vi "SMUSineWithReferenceTrigger.vi"() -> ()   [LabVIEW 2023]
uses:
  <instrlib>/niDCPower/nidcpower.llb/niDCPower Source Mode.ctl
  <instrlib>/niDCPower/nidcpower.llb/niDCPower Output Function.ctl
  <instrlib>/niDCPower/nidcpower.llb/niDCPower Sequence Attribute Type.ctl
  <instrlib>/niDCPower/nidcpower.llb/niDCPower Create Advanced Sequence Step With Channels.vi
  <instrlib>/niScope/Measurements/niScope Fetch Array Measurement Cluster.vi
  <instrlib>/niDCPower/nidcpower.llb/niDCPower Export Signal - Signal.ctl
  <instrlib>/niScope/Configure/Trigger/niScope Configure Trigger Digital.vi
  <instrlib>/niScope/Controls/niScope trigger source digital.ctl
  <instrlib>/niScope/Controls/niScope trigger slope.ctl
  <instrlib>/niScope/Controls/niScope vertical coupling.ctl
panel:
  in  "Configure":enum32{"SMU", "Scope"}(tab)
  in  "SMUname":refnum<k15> caption="resource name"
  in  "DC offset":dbl
  in  "Amplitude":dbl
  in  "Frequency":dbl format="%#_6p"
  in  "Samples per Sine":u16
  in  "?":enum32{"Standard Transients", "Custom"}(tab)
  in  "Source:Transient Response":i32(ring)=1041 items=["Slow"=1041, "Normal"=1038, "Fast"=1039, "Custom"=1042]
  in  "Gain Bandwidth":dbl=5000.0
  in  "Pole-Zero Ratio":dbl=0.16
  in  "Compensation Frequency":dbl=50000.0
  in  "Fixed Source Delay of":dbl format="%#_6p"
  in  "Amount of Sine Swings":i32
  out "Apperature Time":dbl format="%#_6p"
  in  "resource name":refnum<k15> caption="Scope Name"
  in  "Scope sample rate":dbl=20000000.0 caption="min sample rate" format="%^.2e"
  in  "number of records":i32=1
  in  "min record length":i32=1000
  in  "vertical coupling":T1=1 items=["AC", "DC", "Ground"]
  in  "channels":string="0"
  out "Stimulus In":cluster{dbl, dbl}[](graph)
  out "SMU Voltage Out":cluster{dbl, dbl}[](graph)
  out "error out":errorcluster
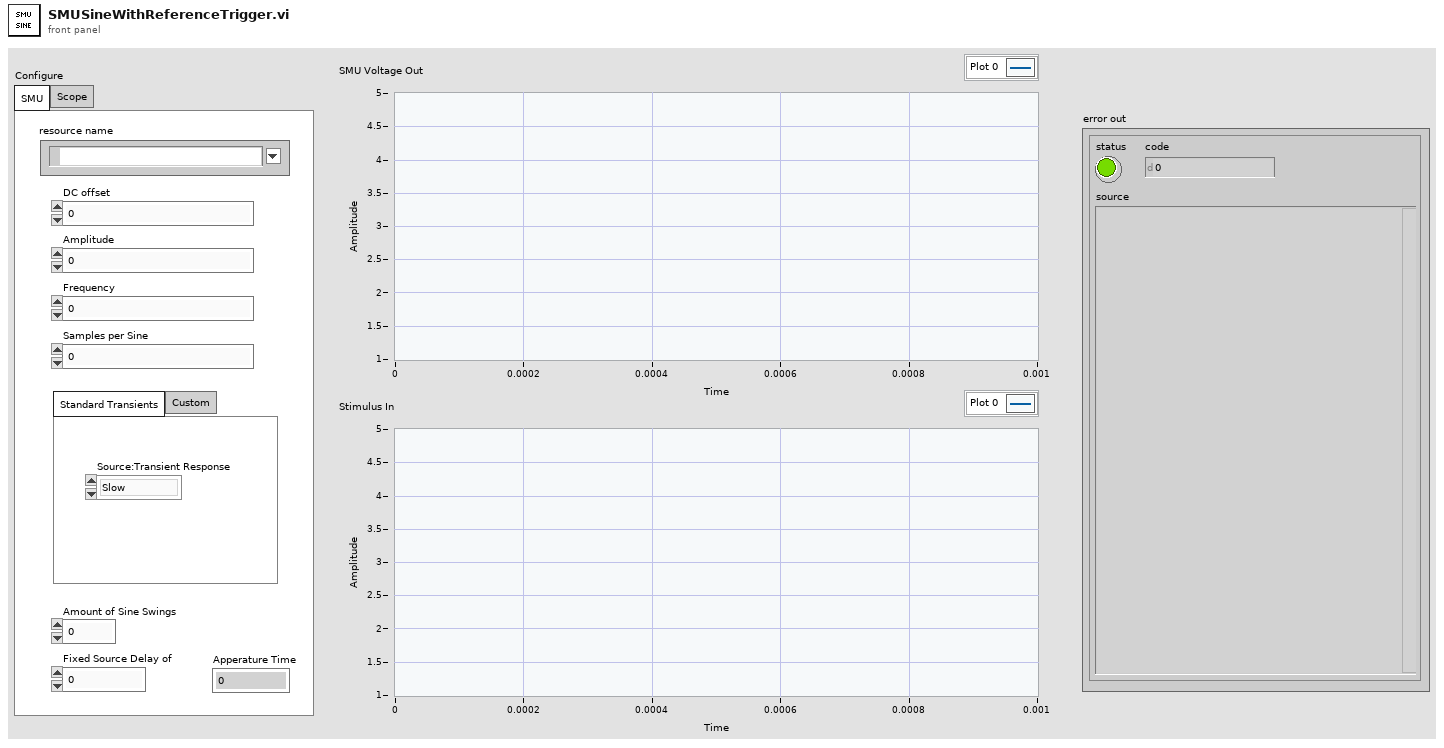
[diagram p1: front panel]
types:
  T1 = typedef "niScope vertical coupling.ctl" = i32
  T2 = typedef "niScope trigger slope.ctl" = i32
  T3 = typedef "niScope trigger source digital.ctl" = string
  T4 = typedef "niDCPower Export Signal - Signal.ctl" = i32
  T5 = typedef "niDCPower Output Function.ctl" = i32
  T6 = typedef "niDCPower Source Mode.ctl" = i32
  T7 = typedef "niDCPower Sequence Attribute Type.ctl" = i32
  T8 = cluster{"relativeInitialX":dbl, "xIncrement":dbl, "measWfm":dbl[]}
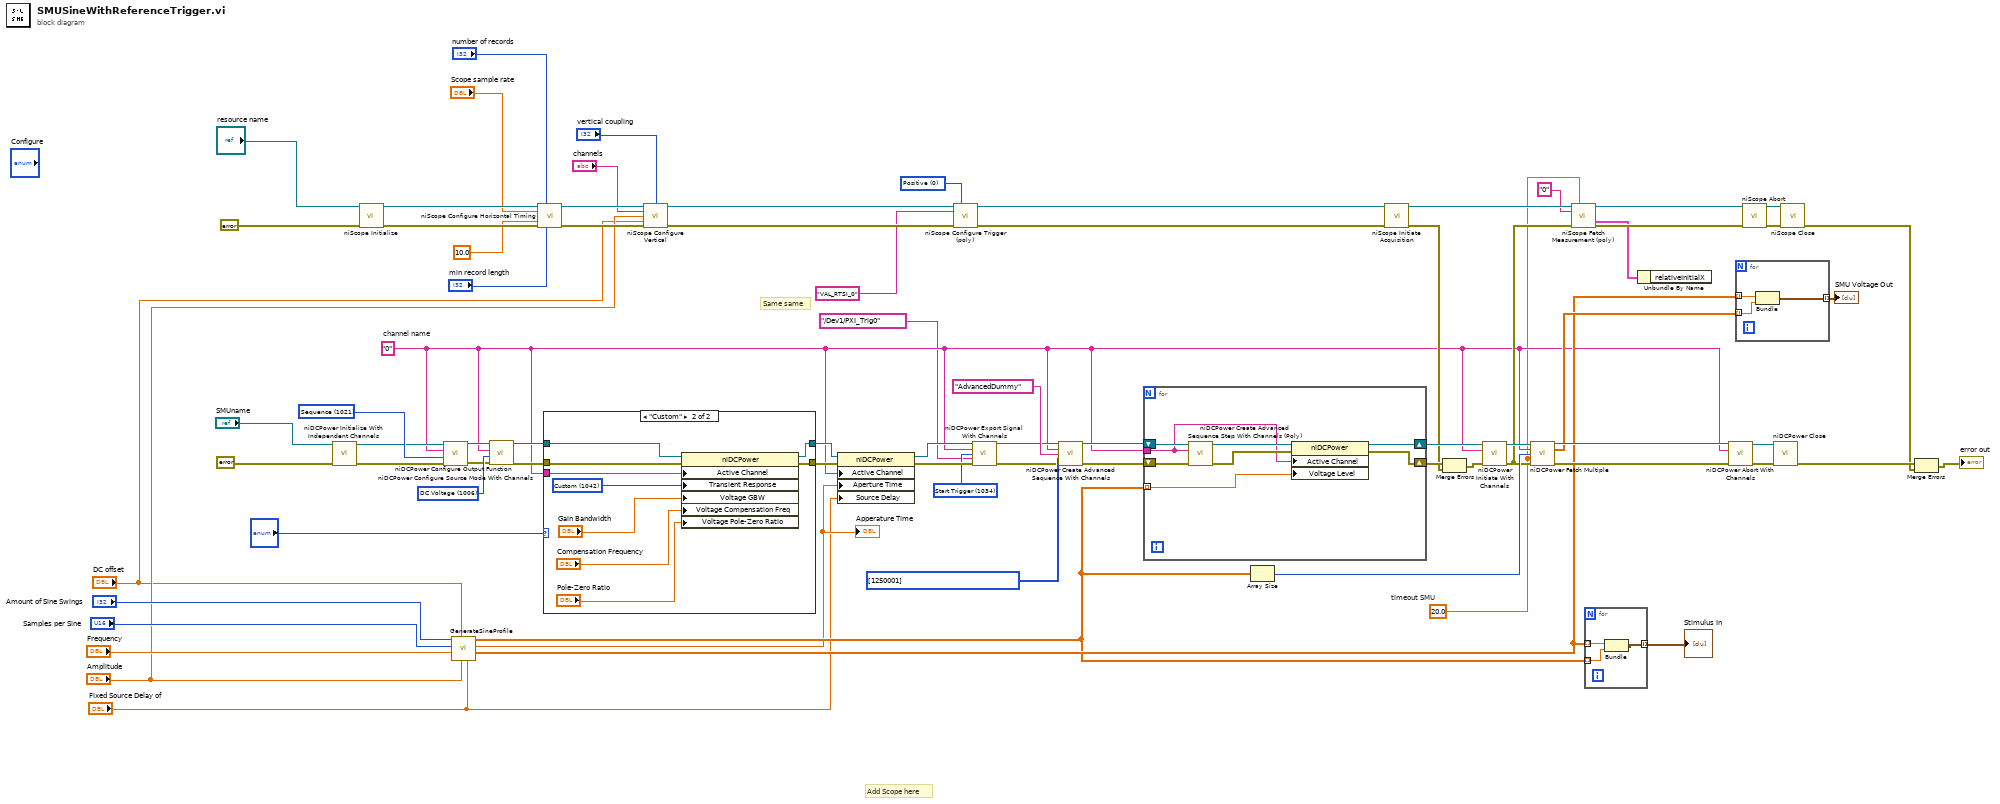
[diagram p0: block diagram]
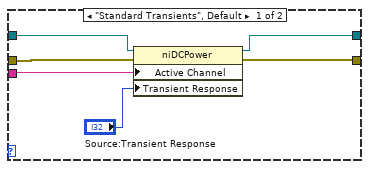
[diagram p2: hidden frame]
diagram:
  w3 = T2 0 items=["Positive", "Negative"] ("trigger slope")
  w6 = T4 1034 items=["Source Complete Event"=1030, "Measure Complete Event"=1031, "Sequence Iteration Complete Event"=1032, "Sequence Engine Done Event"=1033, "Pulse Complete Event"=1051, "Ready For Pulse Trigger Event"=1052, "Start Trigger"=1034, "Source Trigger"=1035, "Measure Trigger"=1036, "Sequence Advance Trigger"=1037, "Pulse Trigger"=1053] ("signal")
  w2 = 20.0  # timeout SMU
  w63 = T5 1006 items=["DC Voltage"=1006, "DC Current"=1007, "Pulse Voltage"=1049, "Pulse Current"=1050] ("output function")
  w66 = T6 1021 items=["Single Point"=1020, "Sequence"=1021] ("source mode")
  w67 = T7[] [1250001] items=["Source -> Output Function"=1150008, "Source -> Output Enabled"=1250006, "Source -> Output Resistance"=1150061, "Source -> Transient Response"=1150062, "Source -> Custom Transient Response -> Voltage Gain Bandwidth"=1150067, "Source -> Custom Transient Response -> Voltage Compensation Frequency"=1150068, "Source -> Custom Transient Response -> Voltage Pole-Zero Ratio"=1150069, "Source -> Custom Transient Response -> Current Gain Bandwidth"=1150070, "Source -> Custom Transient Response -> Current Compensation Frequency"=1150071, "Source -> Custom Transient Response -> Current Pole-Zero Ratio"=1150072, "Source -> DC Voltage -> Voltage Level"=1250001, "Source -> DC Voltage -> Voltage Level Range"=1150005, "Source -> DC Voltage -> Current Limit"=1250005, "Source -> DC Voltage -> Current Limit High"=1150187, "Source -> DC Voltage -> Current Limit Low"=1150188, "Source -> DC Voltage -> Current Limit Range"=1150004, "Source -> DC Current -> Current Level"=1150009, "Source -> DC Current -> Current Level Range"=1150011, "Source -> DC Current -> Voltage Limit"=1150010, "Source -> DC Current -> Voltage Limit High"=1150185, "Source -> DC Current -> Voltage Limit Low"=1150186, "Source -> DC Current -> Voltage Limit Range"=1150012, "Source -> DC Current -> Current Level Slew Rate -> Rising"=1150343, "Source -> DC Current -> Current Level Slew Rate -> Falling"=1150344, "Source -> Pulse Voltage -> Pulse Voltage Level"=1150080, "Source -> Pulse Voltage -> Pulse Bias Voltage Level"=1150082, "Source -> Pulse Voltage -> Pulse Voltage Level Range"=1150084, "Source -> Pulse Voltage -> Pulse Current Limit"=1150081, "Source -> Pulse Voltage -> Pulse Current Limit High"=1150193, "Source -> Pulse Voltage -> Pulse Current Limit Low"=1150194, "Source -> Pulse Voltage -> Pulse Bias Current Limit"=1150083, "Source -> Pulse Voltage -> Pulse Bias Current Limit High"=1150195, "Source -> Pulse Voltage -> Pulse Bias Current Limit Low"=1150196, "Source -> Pulse Voltage -> Pulse Current Limit Range"=1150085, "Source -> Pulse Current -> Pulse Current Level"=1150086, "Source -> Pulse Current -> Pulse Bias Current Level"=1150088, "Source -> Pulse Current -> Pulse Current Level Range"=1150090, "Source -> Pulse Current -> Pulse Voltage Limit"=1150087, "Source -> Pulse Current -> Pulse Voltage Limit High"=1150189, "Source -> Pulse Current -> Pulse Voltage Limit Low"=1150190, "Source -> Pulse Current -> Pulse Bias Voltage Limit"=1150089, "Source -> Pulse Current -> Pulse Bias Voltage Limit High"=1150191, "Source -> Pulse Current -> Pulse Bias Voltage Limit Low"=1150192, "Source -> Pulse Current -> Pulse Voltage Limit Range"=1150091, "Source -> Advanced -> Source Delay"=1150051, "Source -> Advanced -> Pulse Bias Delay"=1150092, "Source -> Advanced -> Pulse On Time"=1150093, "Source -> Advanced -> Pulse Off Time"=1150094, "Source -> Advanced -> OVP Enabled"=1250002, "Source -> Advanced -> OVP Limit"=1250003, "Source -> Advanced -> Compliance Limit Symmetry"=1150184, "Source -> Advanced -> Sequence Step Delta Time"=1150198, "Source -> Advanced -> Conduction Voltage -> Mode"=1150350, "Source -> Advanced -> Conduction Voltage -> On Threshold"=1150351, "Source -> Advanced -> Conduction Voltage -> Off Threshold"=1150352, "Measurement -> Sense"=1150013, "Measurement -> Aperture Time"=1150058, "Measurement -> Measure Record Length"=1150063, "Measurement -> Advanced -> DC Noise Rejection"=1150066, "Measurement -> Autorange"=1150244, "Measurement -> Advanced -> Autorange Behavior"=1150245, "Measurement -> Advanced -> Autorange Aperture Time Mode"=1150246, "Measurement -> Advanced -> Autorange Minimum Aperture Time"=1150247, "Measurement -> Advanced -> Autorange Minimum Aperture Time Units"=1150248, "Measurement -> Advanced -> Autorange Minimum Current Range"=1150255, "Measurement -> Advanced -> Autorange Minimum Voltage Range"=1150256, "Measurement -> Advanced -> Autorange Threshold Mode"=1150257, "Measurement -> Advanced -> Autorange Maximum Delay After Range Change"=1150322, "LCR -> Instrument Mode"=1150208, "LCR -> Source Delay Mode"=1150315, "LCR -> Measurement Time"=1150218, "LCR -> Custom Measurement Time"=1150258, "LCR -> AC Stimulus -> Function"=1150209, "LCR -> AC Stimulus -> Frequency"=1150210, "LCR -> AC Stimulus -> Voltage Amplitude"=1150211, "LCR -> AC Stimulus -> Current Amplitude"=1150212, "LCR -> AC Stimulus -> Advanced -> Voltage Range"=1150265, "LCR -> AC Stimulus -> Advanced -> Current Range"=1150267, "LCR -> AC Stimulus -> Advanced -> Source Aperture Time"=1150349, "LCR -> DC Bias -> Source"=1150213, "LCR -> DC Bias -> Voltage Level"=1150214, "LCR -> DC Bias -> Current Level"=1150215, "LCR -> DC Bias -> Advanced -> Voltage Range"=1150266, "LCR -> DC Bias -> Advanced -> Current Range"=1150274, "LCR -> DC Bias -> Advanced -> Transient Response"=1150347, "LCR -> Compensation -> Open -> Enabled"=1150220, "LCR -> Compensation -> Open -> Conductance"=1150261, "LCR -> Compensation -> Open -> Susceptance"=1150262, "LCR -> Compensation -> Short -> Enabled"=1150221, "LCR -> Compensation -> Short -> Resistance"=1150263, "LCR -> Compensation -> Short -> Reactance"=1150264, "LCR -> Compensation -> Load -> Enabled"=1150222, "LCR -> Compensation -> Load -> Measured Resistance"=1150268, "LCR -> Compensation -> Load -> Measured Reactance"=1150269, "LCR -> Compensation -> Load -> Actual Resistance"=1150270, "LCR -> Compensation -> Load -> Actual Reactance"=1150271, "LCR -> Impedance Range -> Impedance Range"=1150217, "LCR -> Impedance Range -> Impedance Autorange"=1150216, "LCR -> Impedance Range -> Advanced -> Impedance Range Source"=1150321, "LCR -> Impedance Range -> Advanced -> Load Resistance"=1150318, "LCR -> Impedance Range -> Advanced -> Load Inductance"=1150319, "LCR -> Impedance Range -> Advanced -> Load Capacitance"=1150320] ("advanced sequence properties")
  w7 = "0"  # channel name
  # "Same same"
  # "Add Scope here"
  n1 = call <instrlib>:"niDCPower Initialize With Independent Channels.vi"("error in (no error)"=errorcluster {"status"=FALSE, "code"=0, "source"=""}, "resource name"="SMUname") -> ("error out"=w64:errorcluster, "instrument handle out"=w65:refnum<k15>)  [unwired: 8 in]
  n2 = call <instrlib>:"niScope Initialize.vi"("resource name"="resource name", "error in"=errorcluster {"status"=FALSE, "code"=0, "source"=""}) -> ("instrument handle"=w42:refnum<k15>, "error out"=w41:errorcluster)  [unwired: 12 in]
  n3 = call <instrlib>:"niDCPower Configure Source Mode With Channels.vi"("error in (no error)"=w64, "source mode"=w66, "channel name"=w7, "instrument handle"=w65) -> ("error out"=w61:errorcluster, "instrument handle out"=w62:refnum<k15>)  [unwired: 6 in]
  n4 = call "GenerateSineProfile.vi"("Fixed Source Delay of"="Fixed Source Delay of", "Amplitude"="Amplitude", "DC offset"="DC offset", "Frequency"="Frequency", "Samples per Sine"="Samples per Sine", "Amount of Itterations"="Amount of Sine Swings") -> ("Time to Plot"=w49:dbl[], "Apperature Time"=w45:dbl, "Voltage"=w48:dbl[])  [unwired: 3 in]
  "Apperature Time" <- w45
  n5 = call <instrlib>:"niDCPower Configure Output Function.vi"("error in (no error)"=w61, "output function"=w63, "channel name"=w7, "instrument handle"=w62) -> ("error out"=w56:errorcluster, "instrument handle out"=w55:refnum<k15>)  [unwired: 6 in]
  n6 = call <instrlib>:"niScope Configure Horizontal Timing.vi"("instrument handle"=w42, "number of records"="number of records", "min sample rate"="Scope sample rate", "reference position"=10.0, "error in"=w41, "min record length"="min record length") -> ("instrument handle out"=w40:refnum<k15>, "error out"=w39:errorcluster)  [unwired: 8 in]
  n7 = case shown="\"Custom\"" "?" {
    tunnel: [w82 w91] -> w46
    tunnel: w56 -> [w79 w90]
    tunnel: w55 -> [w80 w89]
    tunnel: w7 -> [w78 w88]
    tunnel: [w81 w87] -> w47
    frame "Standard Transients", Default {
      n8 = property class="niDCPower"(reference=w80, error in=w79, "Active Channel"=w78, "Transient Response"="Source:Transient Response") -> (reference out=w81:refnum<k15>, error out=w82:errorcluster)
    }
    frame "Custom" {
      w86 = 1042 items=["Slow"=1041, "Normal"=1038, "Fast"=1039, "Custom"=1042] ("Source:Transient Response")
      n9 = property class="niDCPower"(reference=w89, error in=w90, "Active Channel"=w88, "Transient Response"=w86, "Voltage GBW"="Gain Bandwidth", "Voltage Compensation Freq"="Compensation Frequency", "Voltage Pole-Zero Ratio"="Pole-Zero Ratio") -> (reference out=w87:refnum<k15>, error out=w91:errorcluster)
    }
  }
  n10 = call <instrlib>:"niScope Configure Vertical.vi"("instrument handle"=w40, "vertical coupling"="vertical coupling", "channels"="channels", "vertical range"="Amplitude", "vertical offset"="DC offset", "error in"=w39) -> ("instrument handle out"=w38:refnum<k15>, "error out"=w37:errorcluster)  [unwired: 8 in]
  n11 = property class="niDCPower"(reference=w47, error in=w46, "Active Channel"=w7, "Aperture Time"=w45, "Source Delay"="Fixed Source Delay of") -> (reference out=w9:refnum<k15>, error out=w11:errorcluster)
  n12 = call-poly <instrlib>:"niScope Configure Trigger (poly).vi"("instrument handle"=w38, "trigger slope"=w3, "trigger source"=T3 "VAL_RTSI_0", "error in"=w37) -> ("instrument handle out"=w36:refnum<k15>, "error out"=w35:errorcluster)  [unwired: 10 in]
  n13 = call <instrlib>:"niDCPower Export Signal With Channels.vi"("instrument handle"=w9, "channel name"=w7, "signal"=w6, "output terminal"=tag "/Dev1/PXI_Trig0", "error in (no error)"=w11) -> ("instrument handle out"=w8:refnum<k15>, "error out"=w10:errorcluster)  [unwired: 9 in]
  n14 = call <instrlib>:"niDCPower Create Advanced Sequence With Channels.vi"("instrument handle"=w8, "channel name"=w7, "sequence name"="AdvancedDummy", "advanced sequence properties"=w67, "error in (no error)"=w10) -> ("instrument handle out"=w57:refnum<k15>, "error out"=w58:errorcluster)  [unwired: 9 in]
  n15 = for {
    tunnel: w7 -> [w93]
    shift-right: [w94] -> w74
    shift-left: w57 -> [w99]
    shift-right: [w95] -> w28
    shift-left: w58 -> [w98]
    tunnel: w48 -> [w92] mode=indexing
    n16 = call-poly <instrlib>:"niDCPower Create Advanced Sequence Step With Channels (Poly).vi"("error in (no error)"=w98, "channel name"=w93, "instrument handle"=w99) -> ("error out"=w97:errorcluster, "instrument handle out"=w96:refnum<k15>)  [unwired: 7 in]
    n17 = property class="niDCPower"(reference=w96, error in=w97, "Active Channel"=w93, "Voltage Level"=w92) -> (reference out=w94:refnum<k15>, error out=w95:errorcluster)
  }
  n18 = Array Size(array=w48) -> (size(s)=w60:i32)
  n19 = call <instrlib>:"niScope Initiate Acquisition.vi"("instrument handle"=w36, "error in"=w35) -> ("instrument handle out"=w34:refnum<k15>, "error out"=w27:errorcluster)  [unwired: 12 in]
  n20 = Merge Errors(w28, w27) -> (w29:errorcluster)
  n21 = call <instrlib>:"niDCPower Initiate With Channels.vi"("error in (no error)"=w29, "channel name"=w7, "instrument handle"=w74) -> ("error out"=w26:errorcluster, "instrument handle out"=w73:refnum<k15>)  [unwired: 7 in]
  n22 = call <instrlib>:"niDCPower Fetch Multiple.vi"("instrument handle"=w73, "channel name"=w7, "count (1)"=w60, "timeout (1.0)"=w2, "error in (no error)"=w26) -> ("instrument handle out"=w76:refnum<k15>, "voltage measurements"=w53:dbl[], "error out"=w75:errorcluster)  [unwired: 5 in, 3 out]
  n23 = call-poly <instrlib>:"niScope Fetch Measurement (poly).vi"("instrument handle"=w34, "timeout"=w2, "channels"="0", "error in"=w26) -> ("instrument handle out"=w33:refnum<k15>, "meas waveform"=w20:T8, "error out"=w32:errorcluster)  [unwired: 8 in, 1 out]
  n24 = for {
    tunnel: w49 -> [w102] mode=indexing
    tunnel: w48 -> [w101] mode=indexing
    tunnel: [w100] -> w50 mode=indexing
    n25 = Bundle(w102, w101) -> (w100:cluster{dbl, dbl})  [unwired: 1 in]
  }
  "Stimulus In" <- w50
  n26 = Unbundle By Name(w20) -> ()  [unwired: 1 out]
  n27 = call <instrlib>:"niDCPower Abort With Channels.vi"("error in (no error)"=w75, "channel name"=w7, "instrument handle"=w76) -> ("error out"=w71:errorcluster, "instrument handle out"=w72:refnum<k15>)  [unwired: 7 in]
  n28 = for {
    tunnel: w49 -> [w105] mode=indexing
    tunnel: w53 -> [w104] mode=indexing
    tunnel: [w103] -> w52 mode=indexing
    n29 = Bundle(w105, w104) -> (w103:cluster{dbl, dbl})  [unwired: 1 in]
  }
  "SMU Voltage Out" <- w52
  n30 = call <instrlib>:"niScope Abort.vi"("instrument handle"=w33, "error in"=w32) -> ("instrument handle out"=w31:refnum<k15>, "error out"=w30:errorcluster)  [unwired: 12 in]
  n31 = call <instrlib>:"niDCPower Close.vi"("error in (no error)"=w71, "instrument handle"=w72) -> ("error out"=w25:errorcluster)  [unwired: 9 in]
  n32 = call <instrlib>:"niScope Close.vi"("instrument handle"=w31, "error in"=w30) -> ("error out"=w24:errorcluster)  [unwired: 13 in]
  n33 = Merge Errors(w25, w24) -> (→"error out":errorcluster)
